vi "TPulse.vi"(5 "trigger":bool, 7 "Reset":bool, 9 "TPulse":i32, 11 "error in":errorcluster) -> (6 "Elapsed Time Text":string, 8 "output":bool, 15 "error out":errorcluster)   [LabVIEW 2022 SP3]
uses:
  <vilib>/functionblocks/Edge Detection/Edge Detect/Edge Detect.vi
  <vilib>/functionblocks/FB Core/FB Core.xnode
  <vilib>/functionblocks/NI_FunctionBlock Libraries.lvlib
panel:
  out "Reset elapsed":bool=TRUE caption="Auto Reset"
  out "detected":bool
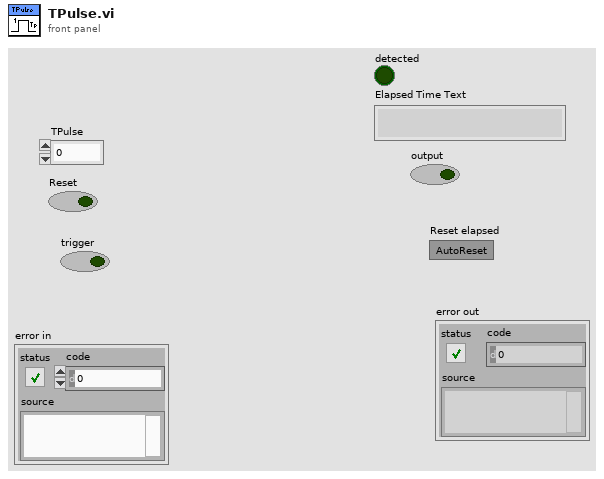
[diagram p1: front panel]
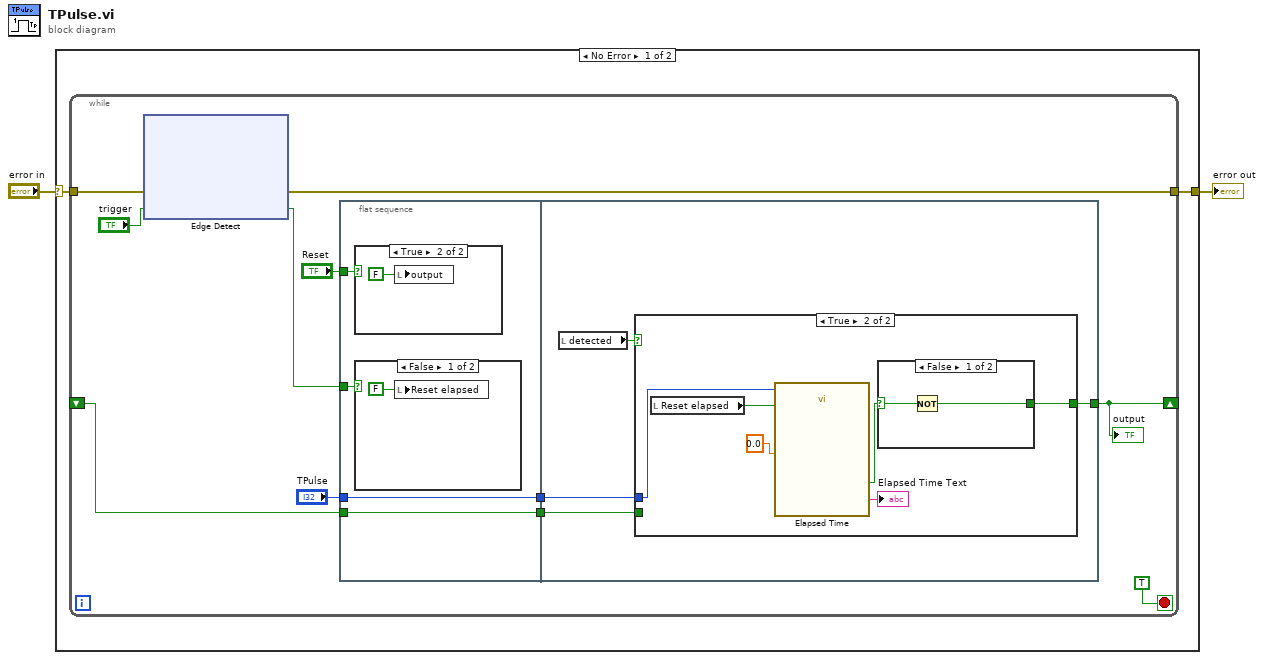
[diagram p0: block diagram]
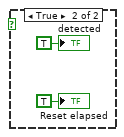
[diagram p3: hidden frame]
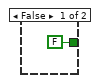
[diagram p4: hidden frame]
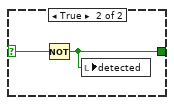
[diagram p5: hidden frame]
diagram:
  n1 = case shown="No Error" "error in" {
    selector: "error in" -> [w4 w84]
    tunnel: [w3 w84] -> w1
    frame No Error {
      n2 = while {
        tunnel: w4 -> [w14]
        tunnel: [w13] -> w3
        shift-right: [w10] -> _
        shift-left: _ -> [w9]
        stop <- TRUE stop-if-true
        n3 = xnode "Edge Detect"("error in"=w14, "input 1"="trigger") -> ("error out"=w13:errorcluster, "output"=w5:bool)
        n4 = flat-sequence {
          tunnel: w9 -> [w18]
          tunnel: "TPulse" -> [w19]
          tunnel: [w19] -> w7
          tunnel: [w18] -> w6
          tunnel: w5 -> [w17]
          tunnel: "Reset" -> [w16]
          tunnel: [w25] -> w10
          tunnel: w7 -> [w27]
          tunnel: w6 -> [w26]
          frame #0 {
            n5 = case shown="True" w16 {
              frame False {
              }
              frame True {
                n6 = local write "output"(FALSE ("output")) -> ()
              }
            }
            n7 = case shown="False" w17 {
              frame False {
                n8 = local write "Reset elapsed"(FALSE ("Reset elapsed")) -> ()
              }
              frame True {
                "detected" <- TRUE ("detected")
                "Reset elapsed" <- TRUE ("Auto Reset")
              }
            }
          }
          frame #1 {
            n9 = local read "detected"() -> (w24:bool)
            n10 = case shown="True" w24 {
              tunnel: w27 -> [_ w34]
              tunnel: [FALSE w32] -> w25
              tunnel: w26 -> [_ _]
              frame False {
              }
              frame True {
                n11 = local read "Reset elapsed"() -> (w29:bool)
                n12 = call "Elapsed Time"("Time Target (s)"=w34, "Reset"=w29, "Set Start Time (s)"=0.0) -> ("Time has Elapsed"=w33:bool, "Elapsed Time Text"=→"Elapsed Time Text":string)  [unwired: 9 in, 6 out]
                n13 = case shown="False" w33 {
                  selector: w33 -> [w36 w38]
                  tunnel: [w35 w37] -> w32
                  frame False {
                    n14 = Not(x=w36) -> (.not. x?=w35:bool)
                  }
                  frame True {
                    n15 = Not(x=w38) -> (.not. x?=w37:bool)
                    n16 = local write "detected"(w37) -> ()
                  }
                }
              }
            }
          }
        }
        "output" <- w10
      }
    }
    frame Error {
    }
  }
  "error out" <- w1
